vi "Read.vi"(7 "LogSuspend":bool, 8 "error in (no error)":errorcluster, 10 "Request Number of Message":i32, 11 "GenericCanAdapterClass in":refnum<class "GenericCanAdapterClass.lvclass">) -> (0 "error out":errorcluster, 2 "Messages":T1[](array[typedef]) {"Data" format="%02x"; "Arbitration Id" format="%03x"}, 3 "GenericCanAdapterClass out":refnum<class "GenericCanAdapterClass.lvclass">)   [LabVIEW 2011, in "GenericCanAdapterClass.lvclass"]
uses:
  GenericCanAdapterClass.lvclass
  National Instruments USB-8473 Adapter/MessageType.ctl
  Private/LogCanRxMessage.vi
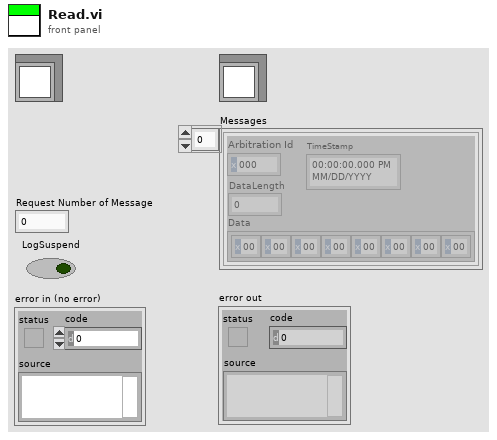
[diagram p1: front panel]
types:
  T1 = typedef "GenericCanAdapterClass.lvclass/MessageType.ctl" = cluster{"Arbitration Id":u32, "Data":u8[], "DataLength":u16, "TimeStamp":timestamp}
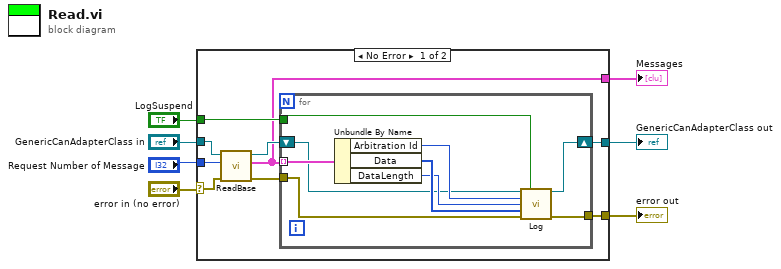
[diagram p0: block diagram]
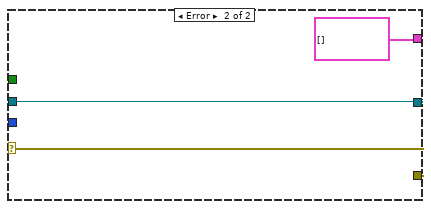
[diagram p2: hidden frame]
diagram:
  n1 = case shown="No Error" "error in (no error)" {
    selector: "error in (no error)" -> [w10 w28]
    tunnel: [w13 w28] -> w4
    tunnel: "GenericCanAdapterClass in" -> [w11 w27]
    tunnel: [w9 w27] -> w2
    tunnel: "LogSuspend" -> [w16 _]
    tunnel: "Request Number of Message" -> [w12 _]
    tunnel: [w8 T1[] [] ("Messages")] -> w1
    frame No Error {
      n2 = call-dynamic "ReadBase.vi"("error in (no error)"=w10, "Request Number of Message"=w12, "GenericCanAdapterClass in"=w11) -> ("error out"=w15:errorcluster, "Messages"=w8:T1[], "GenericCanAdapterClass out"=w14:refnum<class "GenericCanAdapterClass.lvclass">)  [unwired: 6 in]
      n3 = for {
        tunnel: w15 -> [w23]
        tunnel: [w24] -> w13
        tunnel: w8 -> [w25] mode=indexing
        shift-right: [w17] -> w9
        shift-left: w14 -> [w19]
        tunnel: w16 -> [w18]
        n4 = Unbundle By Name(w25) -> ("Arbitration Id"=w20:u32, "Data"=w22:u8[], "DataLength"=w21:u16)
        n5 = call-poly "Log.vi"("GenericCanAdapterClass in"=w19, "LogSuspend"=w18, "Arbitration Id"=w20, "DataLength"=w21, "Data"=w22, "error in"=w23) -> ("GenericCanAdapterClass out"=w17:refnum<class "GenericCanAdapterClass.lvclass">, "error out"=w24:errorcluster)  [unwired: 8 in]
      }
    }
    frame Error {
    }
  }
  "GenericCanAdapterClass out" <- w2
  "error out" <- w4
  "Messages" <- w1
